vi "Start Stop.vi"(0 "VISA resource name":refnum<visa-resource-name>, 5 "Start/Stop (F: Stop)":bool, 11 "error in (no error)":errorcluster) -> (4 "VISA resource name out":refnum<visa-resource-name>, 15 "error out":errorcluster)   [LabVIEW 2013, in "Yokogawa.lvlib" / "Yokogawa PZ4000.lvlib"]
doc: "This VI starts or stops acquisitions; it is functionally identical to pressing the START/STOP button on the instrument's front panel for the PZ4000."
uses:
  Yokogawa PZ4000.lvlib
panel:
  # "Start\nStop"
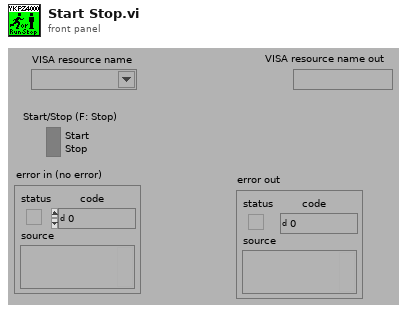
[diagram p1: front panel]
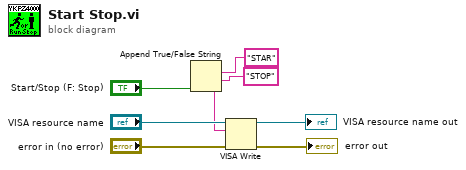
[diagram p0: block diagram]
diagram:
  n1 = Append True/False String(1:"Start/Stop (F: Stop)", 2:"STOP", 3:"STAR") -> (0:w4:string)  [unwired: 1 in]
  n2 = VISA Write(VISA resource name="VISA resource name", write buffer=w4, error in (no error)="error in (no error)") -> (VISA resource name out=→"VISA resource name out":refnum<visa-resource-name>, error out=→"error out":errorcluster)  [unwired: 1 out]
